vi "Calc_Ext.vi"(0 "Reflectivity":dbl[](array[numeric]), 1 "Ambient":dbl[](array[numeric]), 2 "I_zero":dbl[](array[numeric]), 3 "Pressure":dbl, 4 "Temperature":dbl, 6 "Density zero":dbl, 10 "Length_cm":dbl, 11 "Rayleigh zero":dbl[](array[numeric])) -> (22 "Ext":dbl[](array[numeric]))   [LabVIEW 2025]
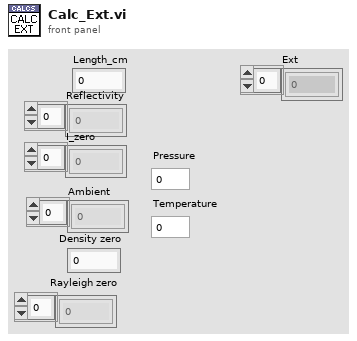
[diagram p1: front panel]
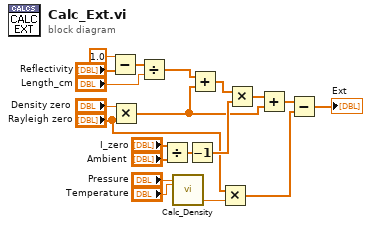
[diagram p0: block diagram]
diagram:
  n1 = Subtract(x=1.0, y="Reflectivity") -> (x-y=w18:dbl[])
  n2 = Multiply(x="Density zero", y="Rayleigh zero") -> (x*y=w6:dbl[])
  n3 = Divide(x=w18, y="Length_cm") -> (x/y=w16:dbl[])
  n4 = Divide(x="I_zero", y="Ambient") -> (x/y=w13:dbl[])
  n5 = call "Calc_Density.vi"("Pres (hPa)"="Pressure", "T (C)"="Temperature") -> ("Density (cm^-3)"=w5:dbl)  [unwired: 25 in]
  n6 = Decrement(x=w13) -> (x-1=w11:dbl[])
  n7 = Add(x=w16, y=w6) -> (x+y=w12:dbl[])
  n8 = Multiply(x="Rayleigh zero", y=w5) -> (x*y=w3:dbl[])
  n9 = Multiply(x=w12, y=w11) -> (x*y=w10:dbl[])
  n10 = Add(x=w10, y=w6) -> (x+y=w4:dbl[])
  n11 = Subtract(x=w4, y=w3) -> (x-y=→"Ext":dbl[])
